vi "FlatToRichnixnet_grpc_DbDeployRequest.vi"(5 "OutputClusterType":T1, 11 "InputCluster":T2) -> (3 "OutputCluster":T1)   [LabVIEW 2025, in "xnet-grpc_client.lvlib"]
uses:
  nixnet_grpc_DbDeployRequest_Flat.ctl
  nixnet_grpc_DbDeployRequest.ctl
  xnet-grpc_client.lvlib
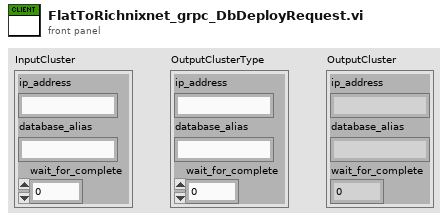
[diagram p1: front panel]
types:
  T1 = typedef "xnet-grpc_client.lvlib/nixnet_grpc_DbDeployRequest.ctl" = cluster{"ip_address":string, "database_alias":string, "wait_for_complete":u32}
  T2 = typedef "xnet-grpc_client.lvlib/nixnet_grpc_DbDeployRequest_Flat.ctl" = cluster{"ip_address":string, "database_alias":string, "wait_for_complete":u32}
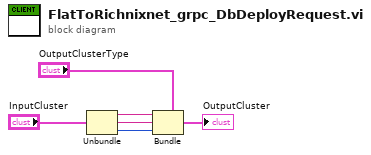
[diagram p0: block diagram]
diagram:
  n1 = Unbundle "Unbundle"("InputCluster") -> ("ip_address"=w3:string, "database_alias"=w2:string, "wait_for_complete"=w1:u32)
  n2 = Bundle "Bundle"(cluster="OutputClusterType", "ip_address"=w3, "database_alias"=w2, "wait_for_complete"=w1) -> (→"OutputCluster":T1)
